vi "占空比测量.vi"(0 "计数器":tag="Dev2/ctr4", 1 "starting edge1":i32(ring)=10280 items=["上升"=10280, "下降"=10171], 2 "starting edge2":i32(ring)=10171 items=["上升"=10280, "下降"=10171], 3 "error in":errorcluster caption="错误输入") -> (7 "占空比(%)":dbl, 8 "占空比2(%)":dbl, 9 "周期(ms)":dbl, 10 "error out":errorcluster caption="错误输出")   [LabVIEW 2020]
uses:
  <vilib>/DAQmx/read.llb/DAQmx Read (Counter 1D DBL 1Chan NSamp).vi
  <vilib>/DAQmx/create/channels.llb/DAQmx Create Channel (CI-Pulse Width).vi
  <vilib>/DAQmx/configure/timing.llb/DAQmx Timing (Implicit).vi
  <vilib>/DAQmx/miscellaneous.llb/DAQmx Fill In Error Info.vi
  <userlib>/_MGI/1D Array/MGI Average/MGI Average (DBL[]).vi
  <resource>/objmgr/daqmx.rc
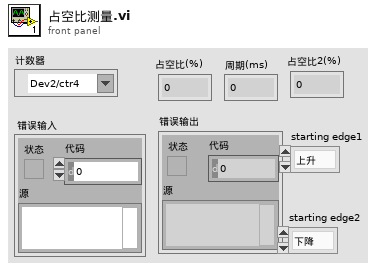
[diagram p1: front panel]
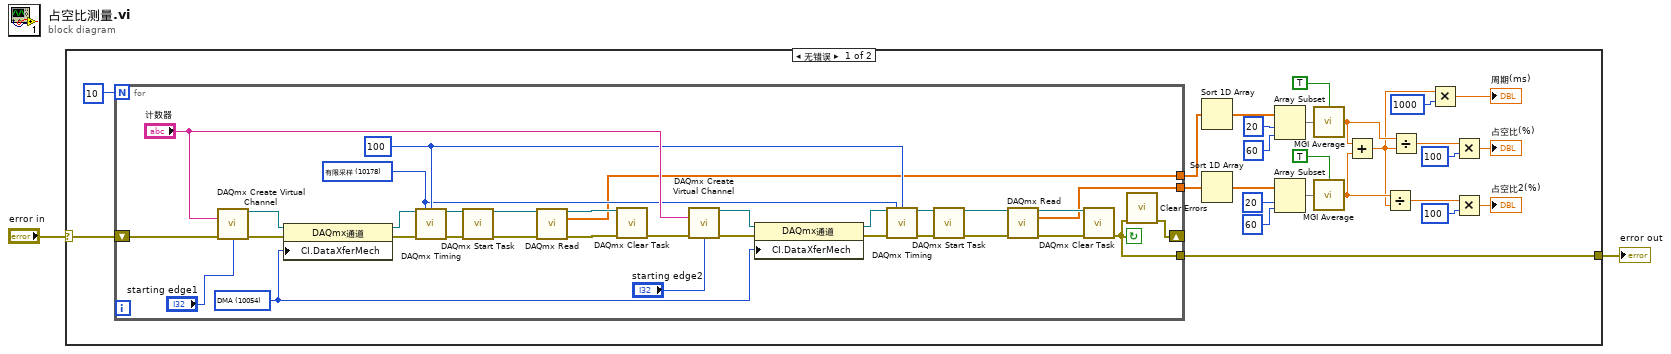
[diagram p0: block diagram]
diagram:
  n1 = case shown="无错误" "error in" {
    selector: "error in" -> [w26 w61]
    tunnel: [w24 w61] -> w1
    frame No Error {
      n2 = for {
        N: 10 -> [_]
        tunnel: [w42] -> w23
        tunnel: [w41] -> w22
        shift-right: [w31] -> _
        shift-left: w26 -> [w40]
        tunnel: [w32] -> w24
        stop <- w32 continue-if-true
        w33 = 10054 items=["DMA"=10054, "中断"=10204, "程序控制I/O"=10264, "USB Bulk"=12590] ("CI.DataXferMech")
        w45 = 100 ("samples per channel")
        w44 = 10178 items=["有限采样"=10178, "连续采样"=10123, "硬件定时单点"=12522] ("sample mode")
        n3 = call-poly <vilib>:"DAQmx Create Virtual Channel.vi"("counter"="计数器", "error in"=w40, "starting edge"="starting edge1") -> ("task out"=w60:refnum<k21>, "error out"=w38:errorcluster)  [unwired: 11 in]
        n4 = property class="DAQmx通道"(reference=w60, error in=w38, "CI.DataXferMech"=w33) -> (reference out=w39:refnum<k21>, error out=w37:errorcluster)
        n5 = call-poly <vilib>:"DAQmx Timing.vi"("task/channels in"=w39, "sample mode"=w44, "samples per channel"=w45, "error in"=w37) -> ("task out"=w59:refnum<k21>, "error out"=w58:errorcluster)  [unwired: 10 in]
        n6 = call <vilib>:"DAQmx Start Task.vi"("task/channels in"=w59, "error in"=w58) -> ("task out"=w57:refnum<k21>, "error out"=w56:errorcluster)  [unwired: 12 in]
        n7 = call-poly <vilib>:"DAQmx Read.vi"("task/channels in"=w57, "error in"=w56) -> ("task out"=w54:refnum<k21>, "data"=w42:dbl[], "error out"=w55:errorcluster)  [unwired: 11 in]
        n8 = call <vilib>:"DAQmx Clear Task.vi"("task in"=w54, "error in"=w55) -> ("error out"=w43:errorcluster)  [unwired: 13 in]
        n9 = call-poly <vilib>:"DAQmx Create Virtual Channel.vi"("counter"="计数器", "error in"=w43, "starting edge"="starting edge2") -> ("task out"=w49:refnum<k21>, "error out"=w35:errorcluster)  [unwired: 11 in]
        n10 = property class="DAQmx通道"(reference=w49, error in=w35, "CI.DataXferMech"=w33) -> (reference out=w36:refnum<k21>, error out=w34:errorcluster)
        n11 = call-poly <vilib>:"DAQmx Timing.vi"("task/channels in"=w36, "sample mode"=w44, "samples per channel"=w45, "error in"=w34) -> ("task out"=w50:refnum<k21>, "error out"=w51:errorcluster)  [unwired: 10 in]
        n12 = call <vilib>:"DAQmx Start Task.vi"("task/channels in"=w50, "error in"=w51) -> ("task out"=w52:refnum<k21>, "error out"=w53:errorcluster)  [unwired: 12 in]
        n13 = call-poly <vilib>:"DAQmx Read.vi"("task/channels in"=w52, "error in"=w53) -> ("task out"=w46:refnum<k21>, "data"=w41:dbl[], "error out"=w47:errorcluster)  [unwired: 11 in]
        n14 = call <vilib>:"DAQmx Clear Task.vi"("task in"=w46, "error in"=w47) -> ("error out"=w32:errorcluster)  [unwired: 13 in]
        n15 = call <vilib>:"Clear Errors.vi"("error in (no error)"=w32) -> ("error out"=w31:errorcluster)  [unwired: 5 in, 1 out]
      }
      n16 = Sort 1D Array(array=w23) -> (sorted array=w21:dbl[])
      n17 = Sort 1D Array(array=w22) -> (sorted array=w17:dbl[])
      n18 = Array Subset(array=w21, index=20 ("索引"), length=60 ("长度")) -> (w7:dbl[])
      n19 = Array Subset(array=w17, index=20 ("索引"), length=60 ("长度")) -> (w6:dbl[])
      n20 = call-poly <userlib>:"MGI Average.vi"("Double[]"=w7, "Ignore NaN? (F)"=TRUE) -> ("Average"=w16:dbl)
      n21 = call-poly <userlib>:"MGI Average.vi"("Double[]"=w6, "Ignore NaN? (F)"=TRUE) -> ("Average"=w10:dbl)
      n22 = Add(x=w16, y=w10) -> (x+y=w5:dbl)
      n23 = Divide(x=w10, y=w5) -> (x/y=w11:dbl)
      n24 = Divide(x=w16, y=w5) -> (x/y=w28:dbl)
      n25 = Multiply(x=w5, y=1000 ("Waveform")) -> (x*y=→"周期(ms)":dbl)
      n26 = Multiply(x=w28, y=100 ("Waveform")) -> (x*y=→"占空比(%)":dbl)
      n27 = Multiply(x=w11, y=100 ("Waveform")) -> (x*y=→"占空比2(%)":dbl)
    }
    frame Error {
    }
  }
  "error out" <- w1
